vi "Send Transfer Group.vi"(5 "Late Count":i32, 7 "Command":T1=enum."Rx", 8 "error in (no error)":errorcluster, 9 "Transfer Group iteration":u64, 10 "Transfer Group ID":u8, 11 "Plugin Interface in":refnum<class "Plugin Interface.lvclass">) -> (0 "error out":errorcluster, 3 "Plugin Interface out":refnum<class "Plugin Interface.lvclass">)   [LabVIEW 2020, in "DSF Core.lvlib" / "Plugin Interface.lvclass"]
uses:
  Plugin Interface.lvclass
  Command Parameters.ctl
  Command.ctl
  Command Data.ctl
  Send Plugin Command.vi
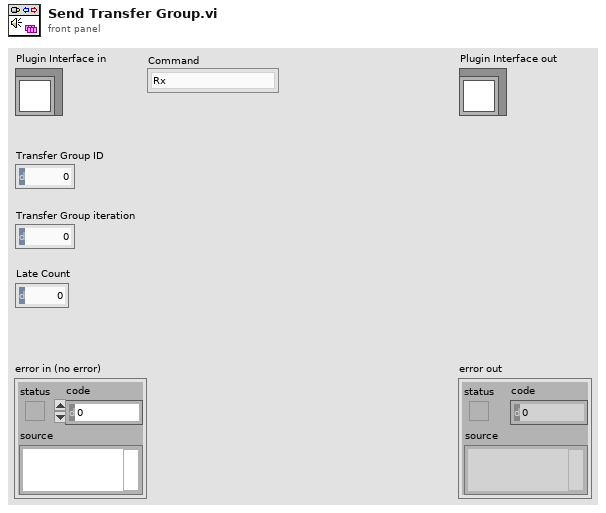
[diagram p1: front panel]
types:
  T1 = typedef "DSF Core.lvlib/Plugin Interface.lvclass/Command.ctl" = enum8{"Idle", "Start", "Set Inline Buffer", "Rx", "Tx", "Shutdown", "Error"}
  T2 = cluster{"Transfer Group ID":i32, "Transfer Group Late Count":i32, "Transfer Group iteration":u64}
  T3 = typedef "DSF Core.lvlib/Plugin Interface.lvclass/Command Parameters.ctl" = cluster{"arg1":u64, "arg2":u64}
  T4 = typedef "DSF Core.lvlib/Plugin Interface.lvclass/Command Data.ctl" = cluster{"Command":T1, "Parameters":T3}
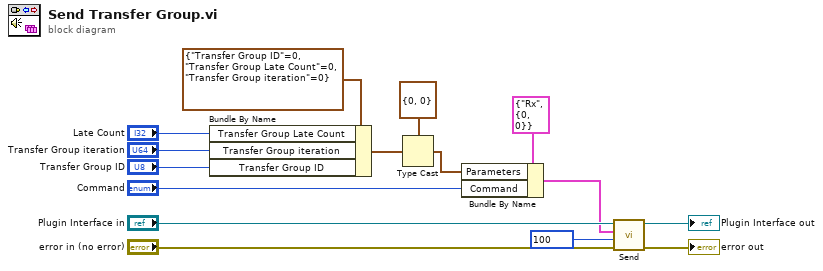
[diagram p0: block diagram]
diagram:
  n1 = Bundle By Name(cluster=T2 {"Transfer Group ID"=0, "Transfer Group Late Count"=0, "Transfer Group iteration"=0}, "Transfer Group Late Count"="Late Count", "Transfer Group iteration"="Transfer Group iteration", "Transfer Group ID"="Transfer Group ID") -> (w11:T2)
  n2 = Type Cast(type=T3 {"arg1"=0, "arg2"=0} ("Command Parameters"), x=w11) -> (*(type *) &x=w13:T3)
  n3 = Bundle By Name(cluster=T4 {"Command"=enum."Rx", "Parameters"={"arg1"=0, "arg2"=0}} ("command"), "Parameters"=w13, "Command"="Command") -> (w3:T4)
  n4 = call-poly "Send.vi"("error in (no error)"="error in (no error)", "timeout in ms (0)"=100, "command"=w3, "Plugin Interface in"="Plugin Interface in") -> ("error out"=→"error out":errorcluster, "Plugin Interface out"=→"Plugin Interface out":refnum<class "Plugin Interface.lvclass">)  [unwired: 6 in]
